vi "Grid_Create Filenames (SubVI).vi"(8 "error in (no error)":errorcluster, 9 "seconds since 1Jan1904":timestamp, 10 "File name":string, 11 "Session path":path) -> (0 "error out":errorcluster, 1 "binFilePath":path, 2 "mainFilePath":path, 3 "Drift File out":refnum<file>, 4 "topoFilePath":path, 5 "zFile":refnum<file>, 7 "xyFile":refnum<file>)   [LabVIEW 2014]
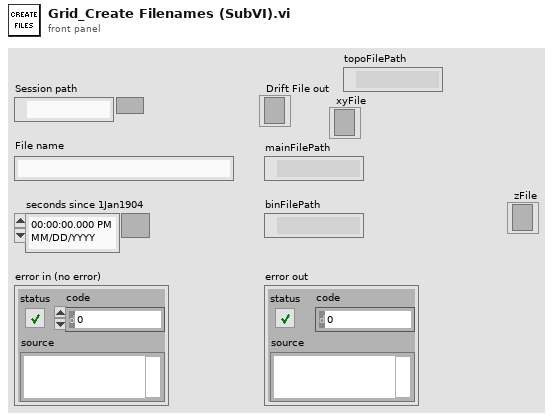
[diagram p1: front panel]
types:
  T1 = enum16{"open", "replace", "create", "open or create", "replace or create", "replace or create with confirmation"}
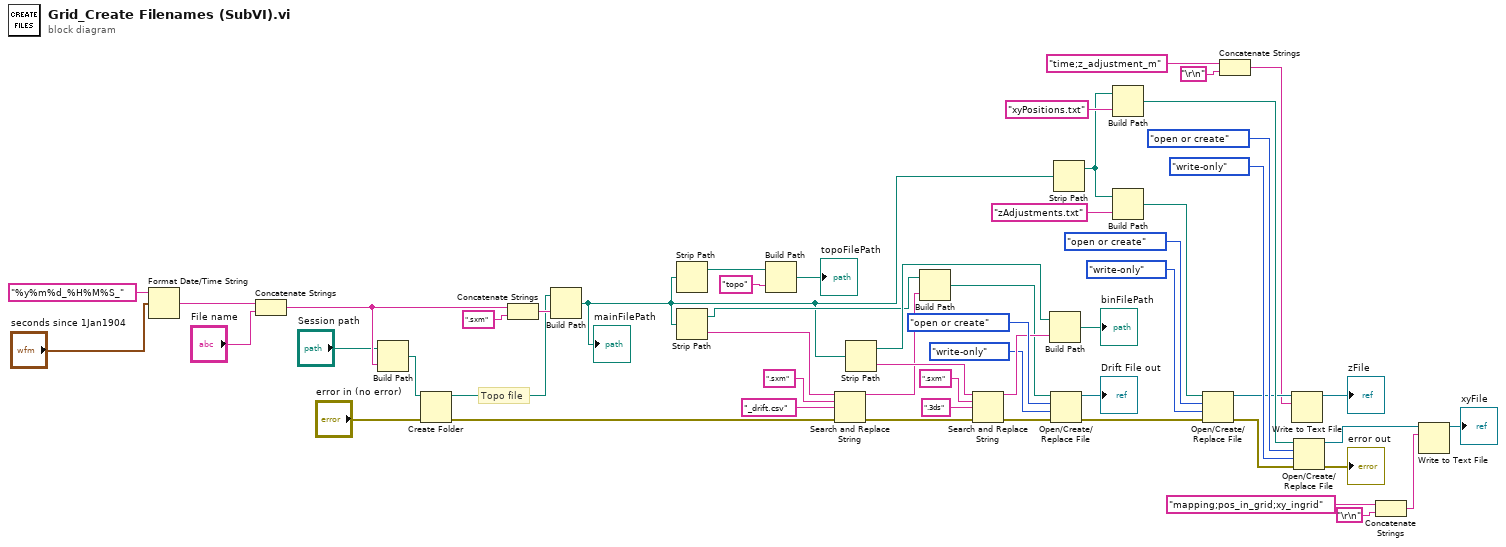
[diagram p0: block diagram]
diagram:
  # "Topo file"
  n1 = Format Date/Time String(time format string (%c)="%y%m%d_%H%M%S_", seconds (now)="seconds since 1Jan1904") -> (date/time string=w52:string)  [unwired: 1 in]
  n2 = Concatenate Strings(w52, "File name") -> (w50:string)
  n3 = Build Path(base path="Session path", name or relative path=w50) -> (appended path=w46:path)
  n4 = Create Folder(path (use dialog)=w46, error in="error in (no error)") -> (created path=w48:path, error out=w13:errorcluster)  [unwired: 1 in, 1 out]
  n5 = Concatenate Strings(w50, ".sxm" ("pattern")) -> (w49:string)
  n6 = Build Path(base path=w48, name or relative path=w49) -> (appended path=w23:path)
  "mainFilePath" <- w23
  n7 = Strip Path(path=w23) -> (stripped path=w25:path)  [unwired: 1 out]
  n8 = Strip Path(path=w23) -> (stripped path=w31:path, name=w34:string)
  n9 = Build Path(base path=w25, name or relative path="topo") -> (appended path=→"topoFilePath":path)
  n10 = Search and Replace String(input string=w34, search string=".sxm", replace string="_drift.csv" ("replace string (\"\")"), error in=w13) -> (result string=w33:string, error out=w12:errorcluster)  [unwired: 4 in, 2 out]
  n11 = Strip Path(path=w23) -> (stripped path=w38:path, name=w39:string)
  n12 = Build Path(base path=w31, name or relative path=w33) -> (appended path=w32:path)
  n13 = Search and Replace String(input string=w39, search string=".sxm", replace string=".3ds" ("replace string (\"\")"), error in=w12) -> (result string=w37:string, error out=w11:errorcluster)  [unwired: 4 in, 2 out]
  n14 = Build Path(base path=w38, name or relative path=w37) -> (appended path=→"binFilePath":path)
  n15 = Open/Create/Replace File(file path (use dialog)=w32, error in=w11, operation (0:open)=T1."open or create", access (0:read/write)=enum16{"read/write", "read-only", "write-only"}."write-only") -> (refnum out=→"Drift File out":refnum<file>, error out=w16:errorcluster)  [unwired: 2 in, 1 out]
  n16 = Strip Path(path=w23) -> (stripped path=w20:path)  [unwired: 1 out]
  n17 = Build Path(base path=w20, name or relative path="xyPositions.txt") -> (appended path=w19:path)
  n18 = Build Path(base path=w20, name or relative path="zAdjustments.txt") -> (appended path=w26:path)
  n19 = Open/Create/Replace File(file path (use dialog)=w26, error in=w16, operation (0:open)=T1."open or create", access (0:read/write)=enum16{"read/write", "read-only", "write-only"}."write-only") -> (refnum out=w4:refnum<file>, error out=w15:errorcluster)  [unwired: 2 in, 1 out]
  n20 = Concatenate Strings("time;z_adjustment_m" ("string"), "\r\n") -> (w2:string)
  n21 = Write to Text File(file (use dialog)=w4, text=w2) -> (refnum out=→"zFile":refnum<file>)  [unwired: 2 in, 2 out]
  n22 = Open/Create/Replace File(file path (use dialog)=w19, error in=w15, operation (0:open)=T1."open or create", access (0:read/write)=enum16{"read/write", "read-only", "write-only"}."write-only") -> (refnum out=w9:refnum<file>, error out=→"error out":errorcluster)  [unwired: 2 in, 1 out]
  n23 = Concatenate Strings("mapping;pos_in_grid;xy_ingrid" ("string"), "\r\n") -> (w8:string)
  n24 = Write to Text File(file (use dialog)=w9, text=w8) -> (refnum out=→"xyFile":refnum<file>)  [unwired: 2 in, 2 out]
